vi "Servo_serial_mac_readwrite2.vi"() -> ()   [LabVIEW 2017]
uses:
  <vilib>/Instr/_visa.llb/VISA Configure Serial Port (Instr).vi
panel:
  out "Servo 5 Torque":cluster{i32, dbl, dbl[]}(graph)
  out "Servo 4 Torque":cluster{i32, dbl, dbl[]}(graph)
  out "Servo 3 Torque":cluster{i32, dbl, dbl[]}(graph)
  out "Servo 2 Torque":cluster{i32, dbl, dbl[]}(graph)
  out "Servo 1 Torque":cluster{i32, dbl, dbl[]}(graph)
  out "case offset":i32
  out "case":string
  out "Torq5 number":dbl
  out "Torq4 number":dbl
  out "Torq3 number":dbl
  out "Torq2 number":dbl
  out "Torq1 number":dbl
  out "Servo 5 Position":cluster{i32, dbl, dbl[][]}(graph)
  out "Servo 4 Position":cluster{i32, dbl, dbl[][]}(graph)
  out "Servo 3 Position":cluster{i32, dbl, dbl[][]}(graph)
  out "Servo 2 Position":cluster{i32, dbl, dbl[][]}(graph)
  out "Servo 1 Position":cluster{i32, dbl, dbl[][]}(graph)
  out "Pos1 number":dbl
  out "Pos2 number":dbl
  out "Pos3 number":dbl
  out "Pos4 number":dbl
  out "Pos5 number":dbl
  in  "Delay":dbl
  in  "Buad Rate":i32(ring) items=["2400"=2400, "4800"=4800, "9600"=9600, "14400"=14400, "19200"=19200, "28800"=28800, "38400"=38400, "57600"=57600, "115200"=115200]
  out "Bytes at port":cluster{i32, dbl, dbl[]}(graph)
  out "Read Buffer":string
  in  "Servo 5":dbl(knob) scale=0.0..180.0
  in  "Servo 4":dbl(knob) scale=0.0..180.0
  in  "Servo 3":dbl(knob) scale=0.0..180.0
  in  "Servo 2":dbl(knob) scale=0.0..180.0
  in  "Servo 1":dbl(knob) scale=0.0..180.0
  in  "stop":bool
  out "Sent to Arduino":string
  in  "COM Port":refnum<visa-resource-name>
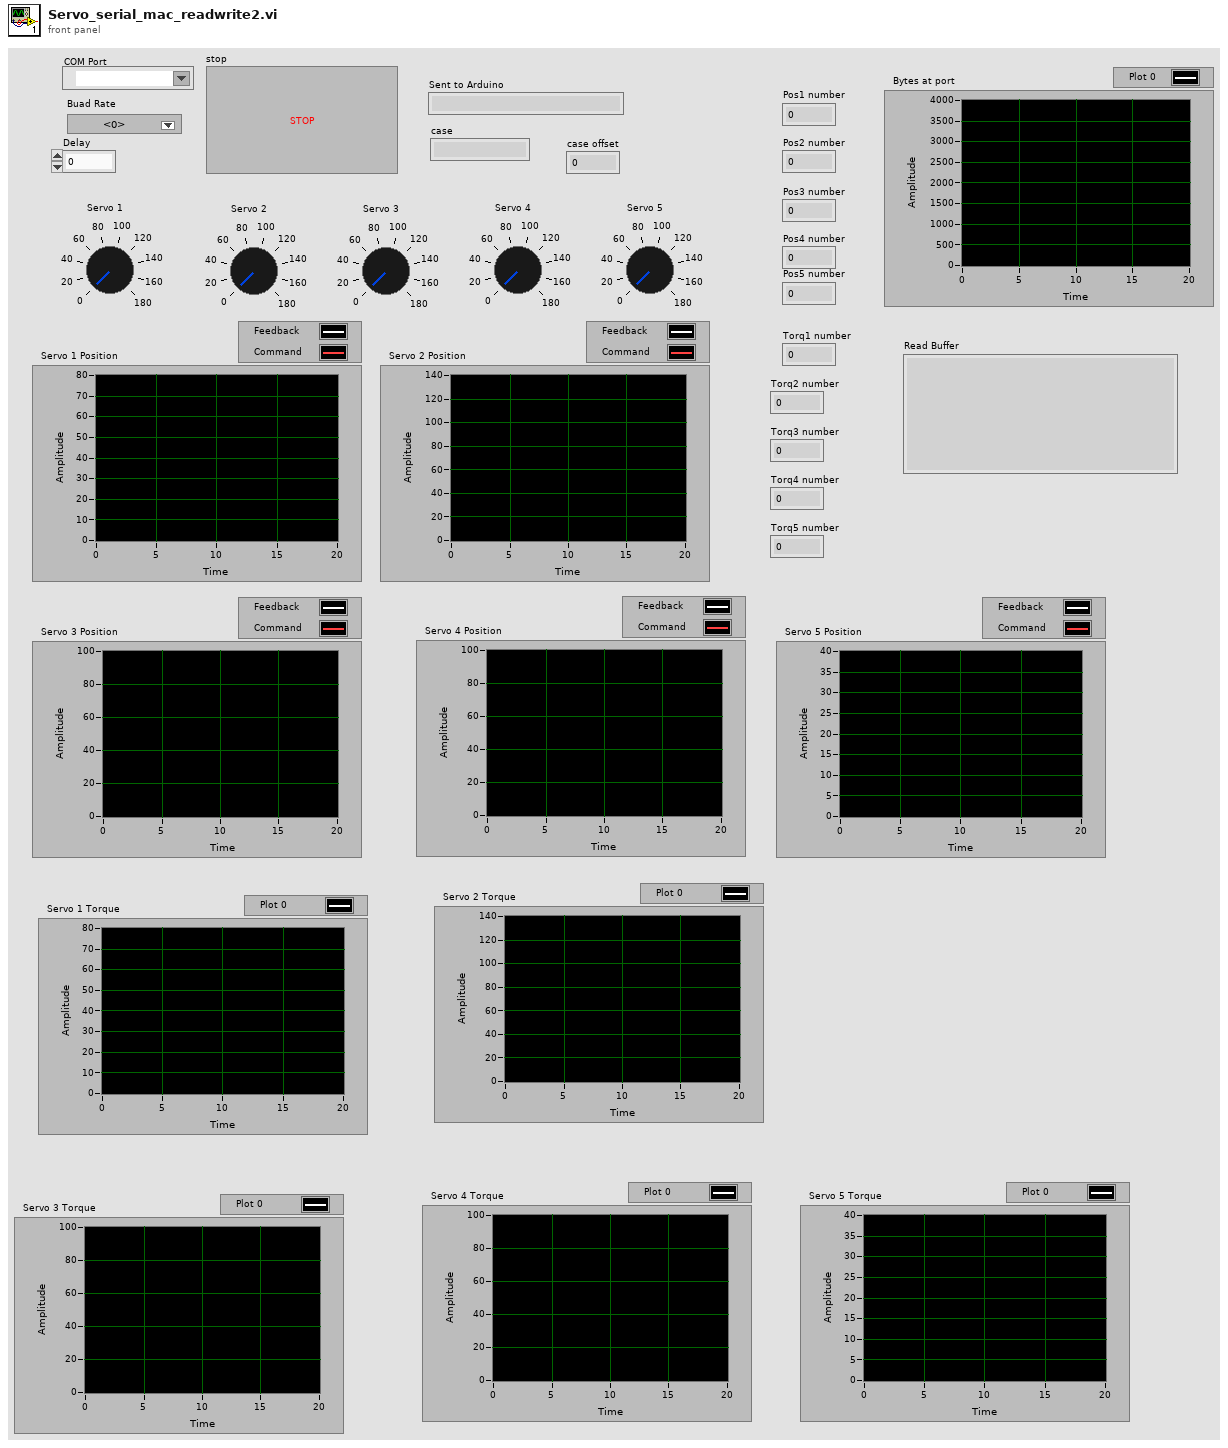
[diagram p1: front panel]
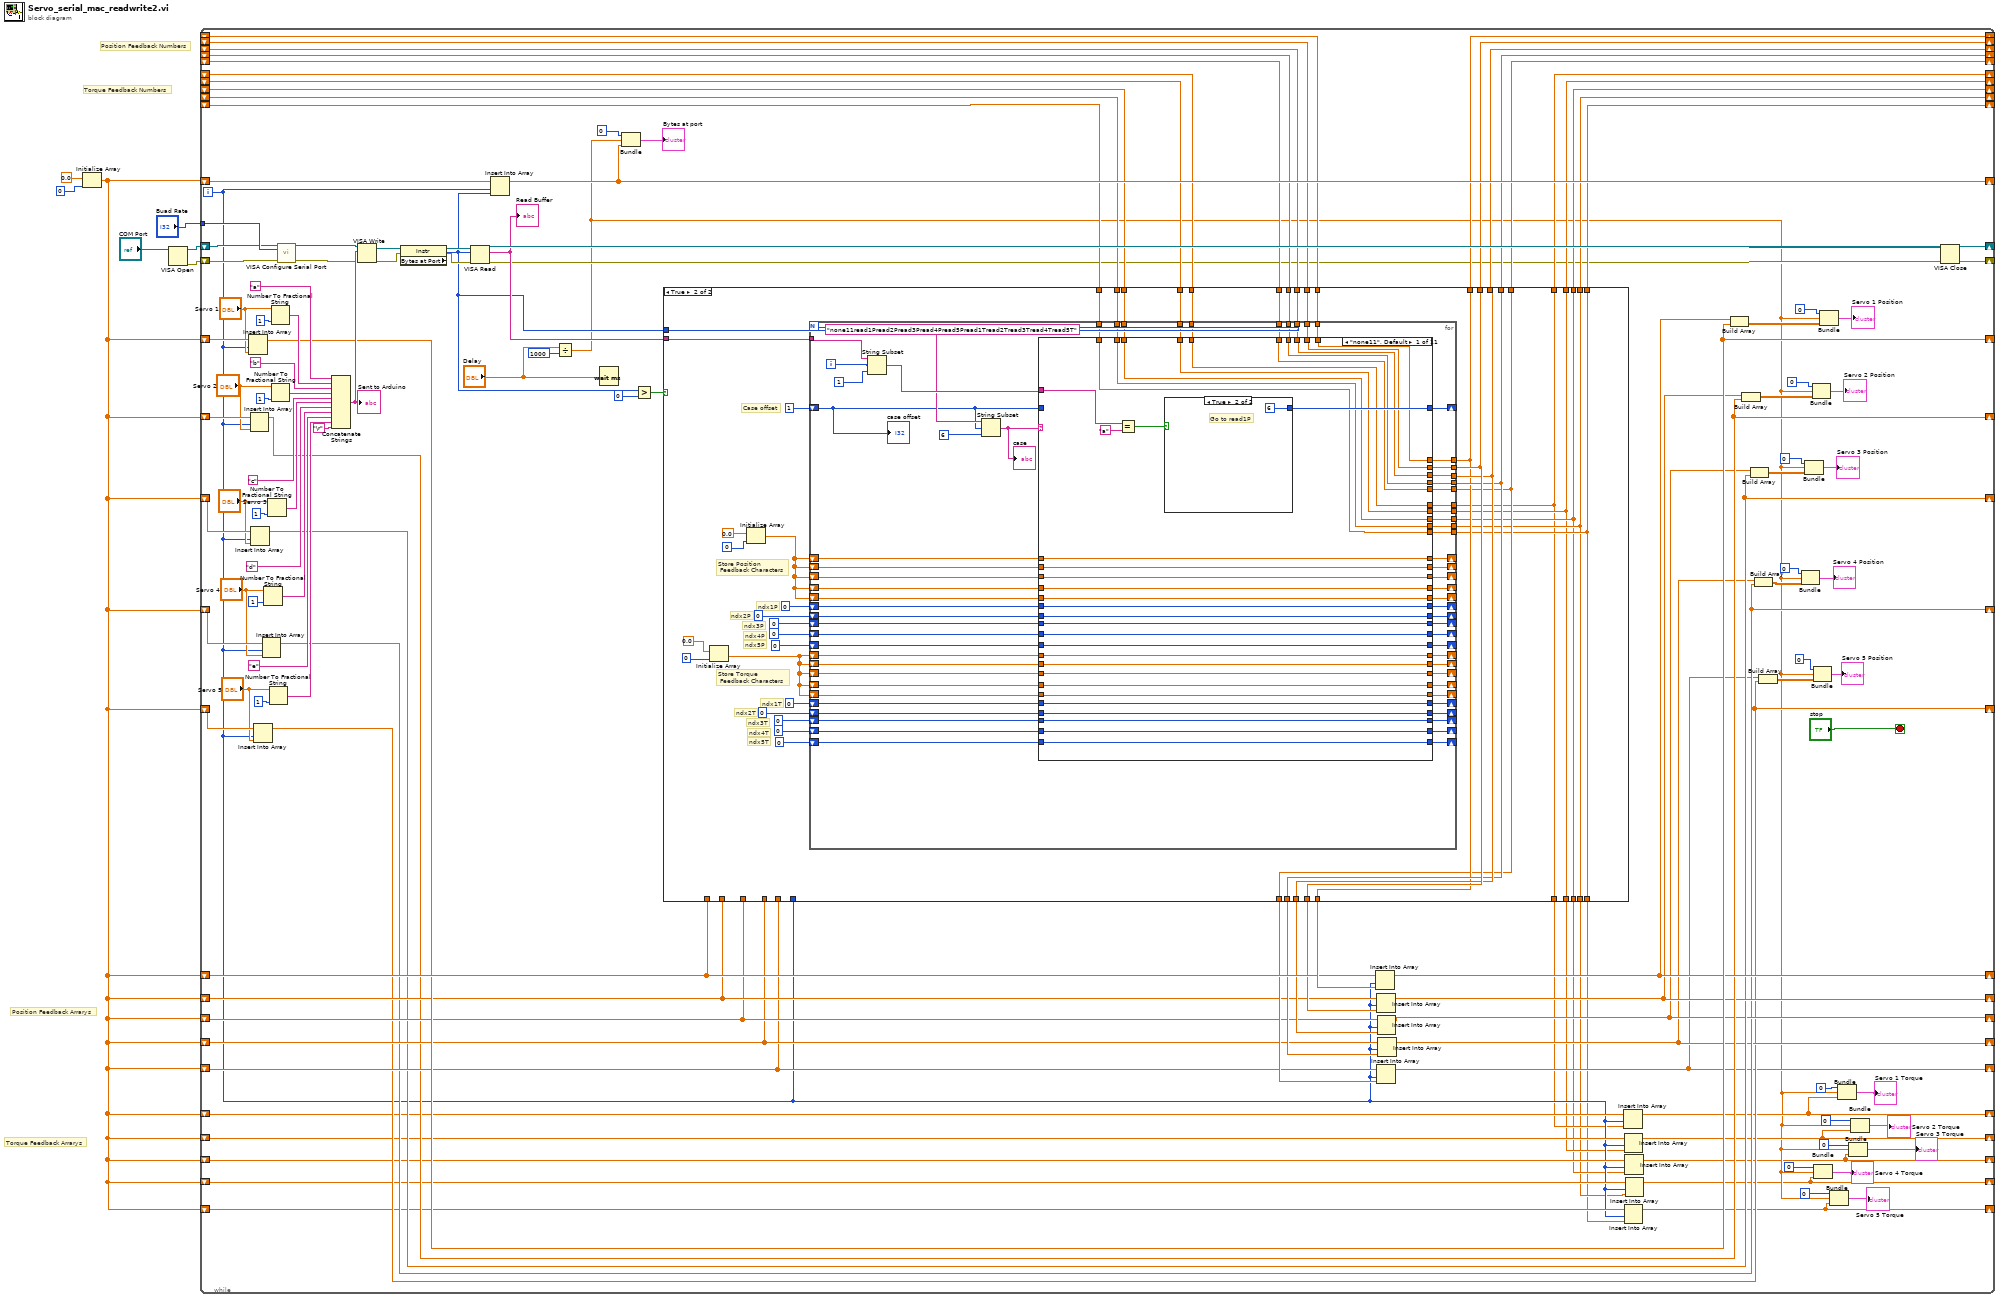
[diagram p0: block diagram]
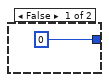
[diagram p3: hidden frame]
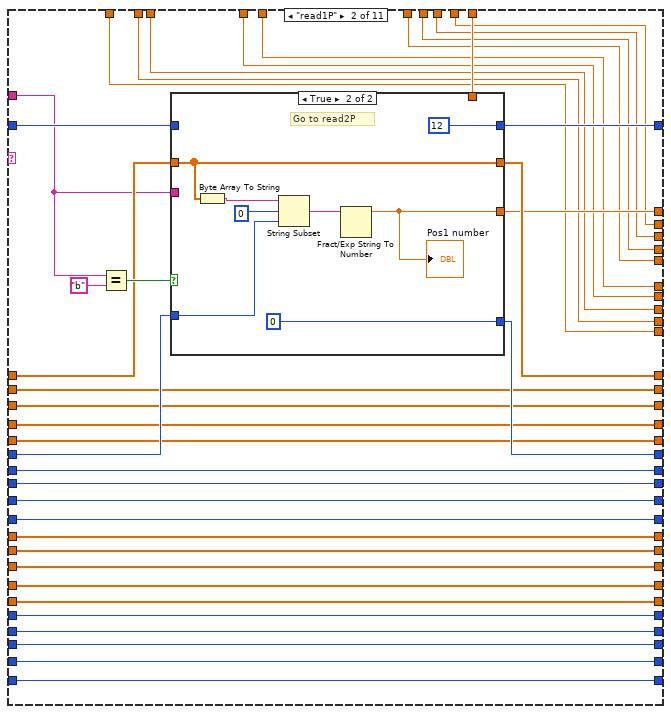
[diagram p4: hidden frame]
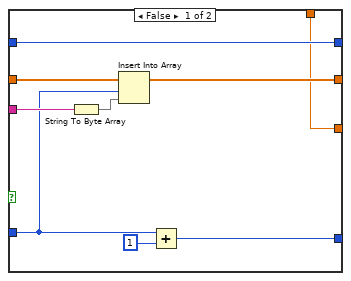
[diagram p5: hidden frame]
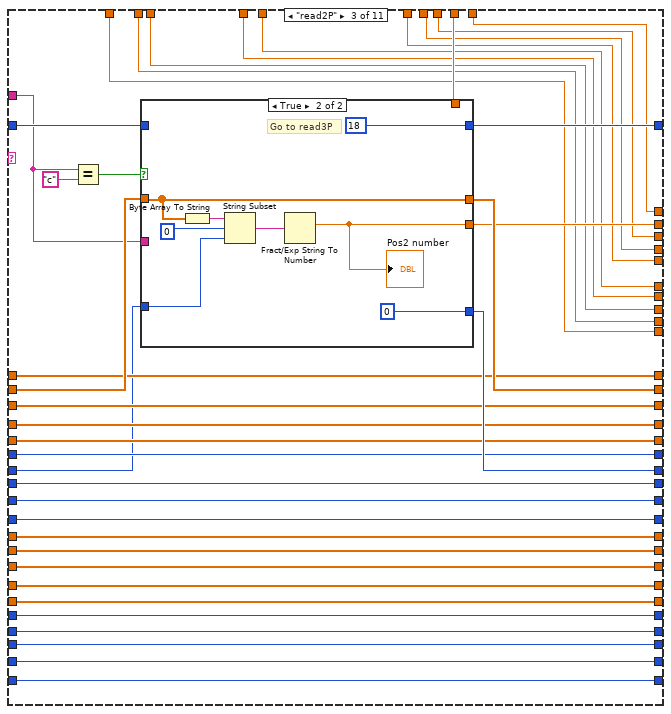
[diagram p6: hidden frame]
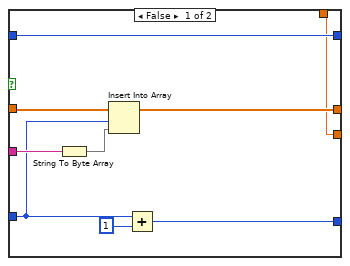
[diagram p7: hidden frame]
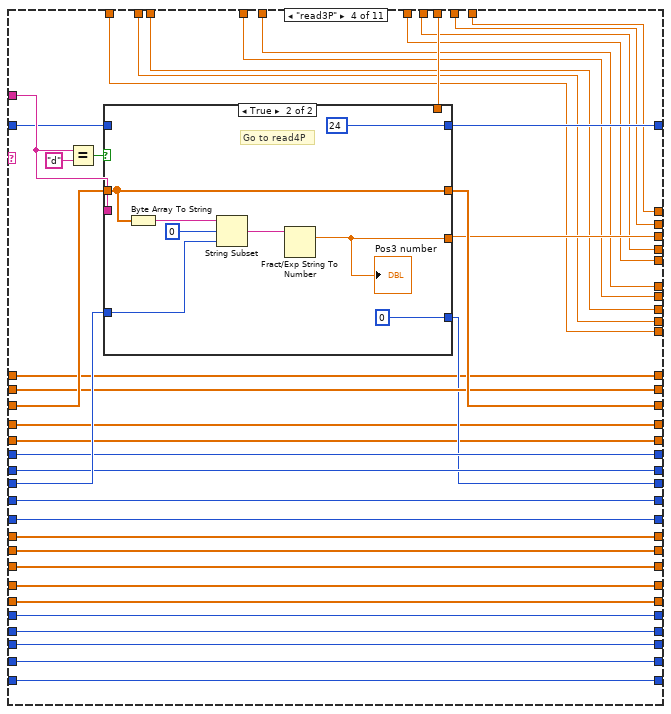
[diagram p8: hidden frame]
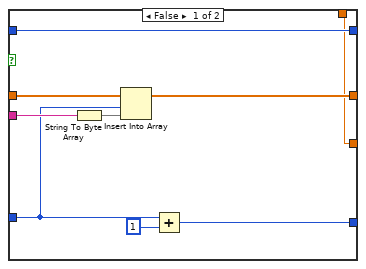
[diagram p9: hidden frame]
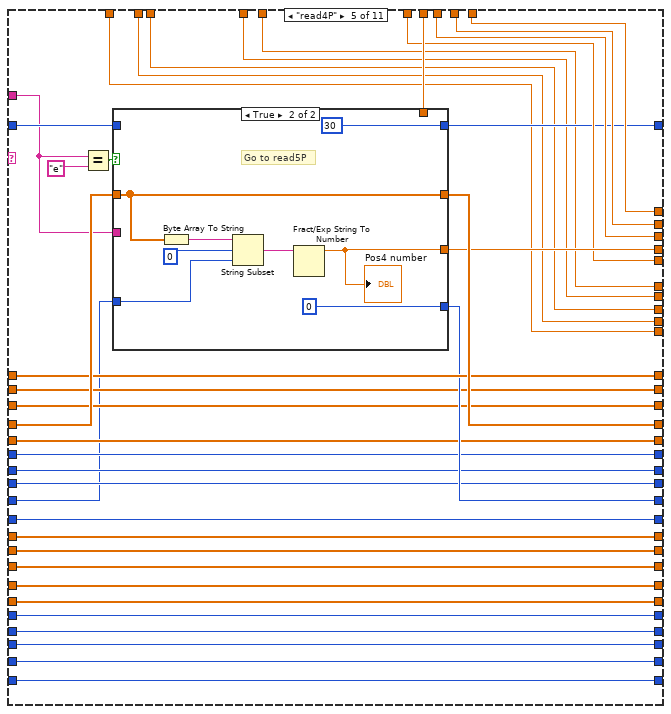
[diagram p10: hidden frame]
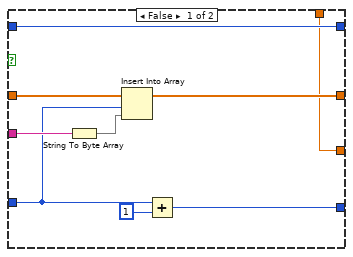
[diagram p11: hidden frame]
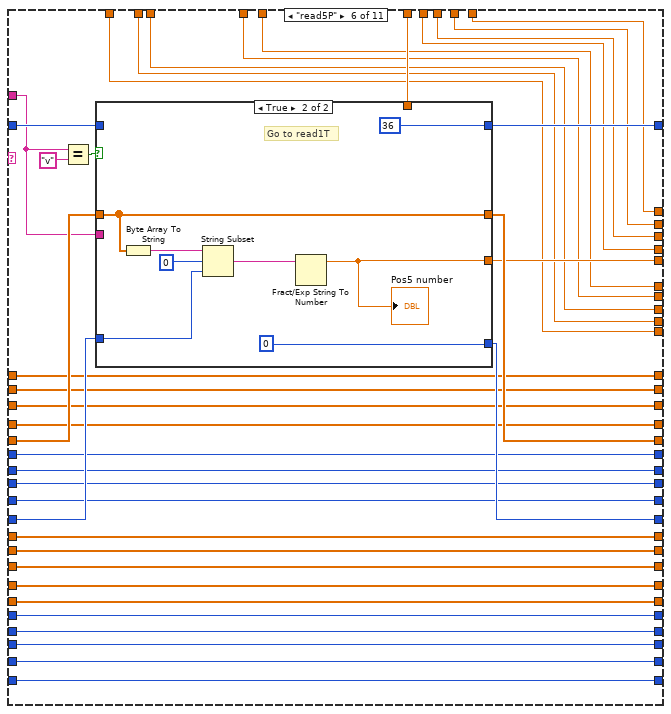
[diagram p12: hidden frame]
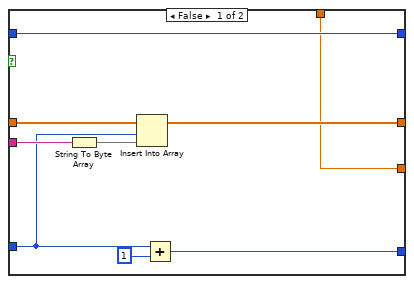
[diagram p13: hidden frame]
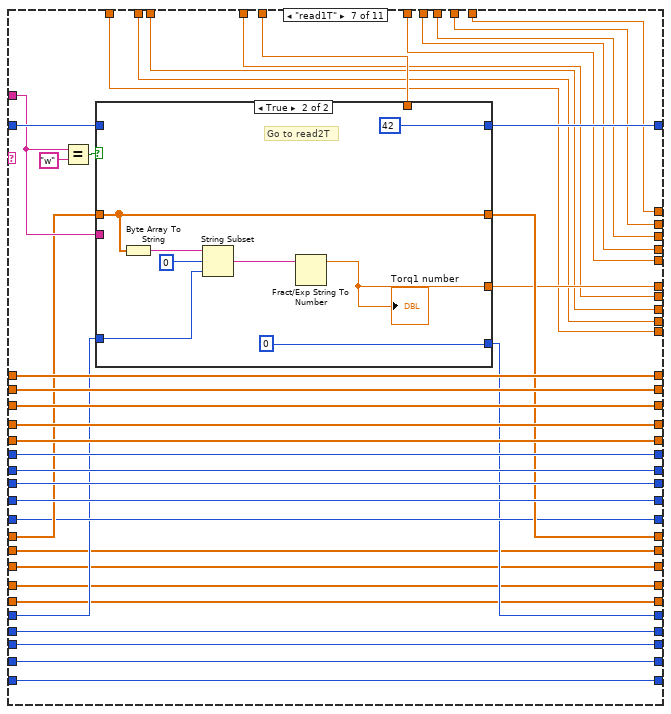
[diagram p14: hidden frame]
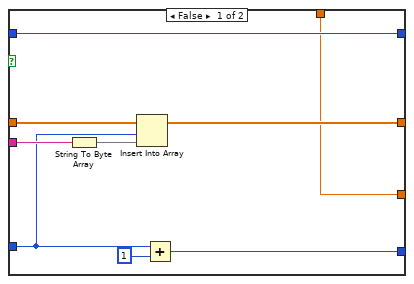
[diagram p15: hidden frame]
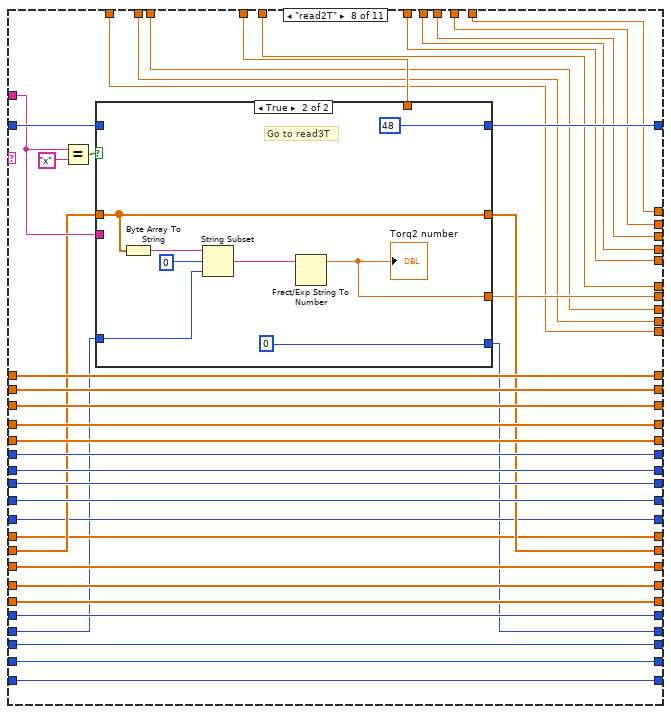
[diagram p16: hidden frame]
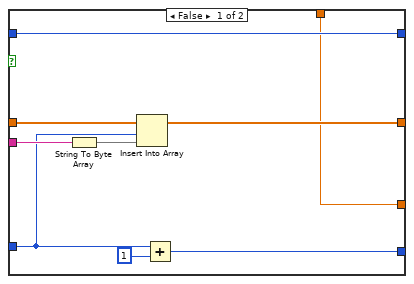
[diagram p17: hidden frame]
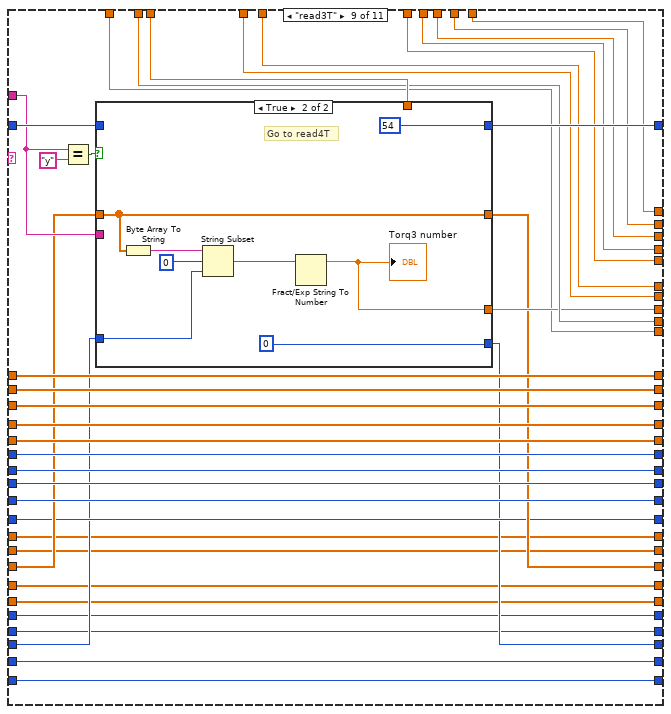
[diagram p18: hidden frame]
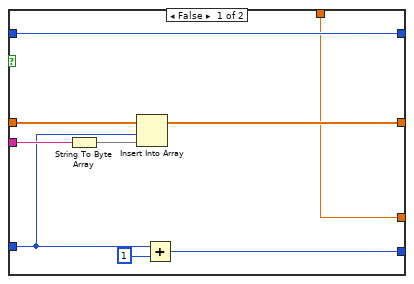
[diagram p19: hidden frame]
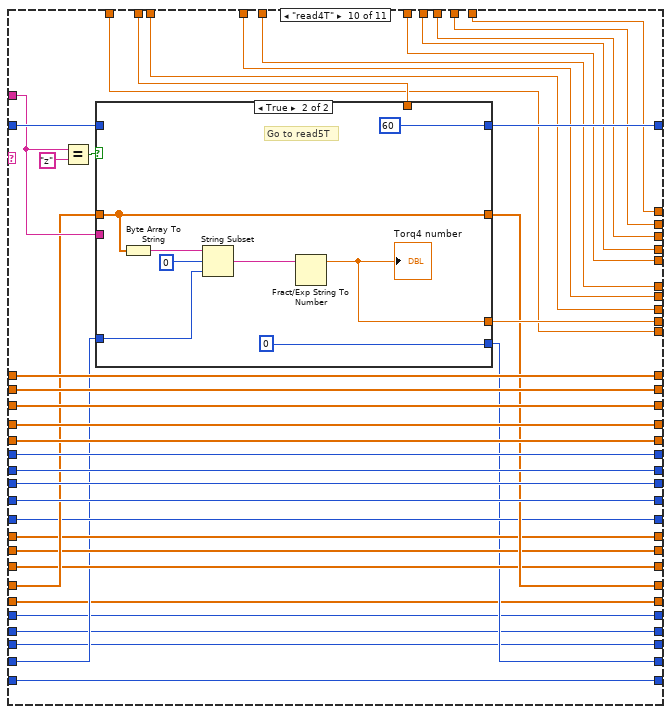
[diagram p20: hidden frame]
diagram:
  # "Torque Feedback Numbers"
  # "Position Feedback Numbers"
  # "Torque Feedback Arrarys"
  # "Position Feedback Arrarys"
  n1 = Initialize Array(0.0 ("element"), 0 ("dimension size")) -> (w1:dbl[])
  n2 = VISA Open(VISA resource name="COM Port") -> (VISA resource name=w8:refnum<visa-resource-name>, error out=w7:errorcluster)  [unwired: 4 in]
  n3 = while {
    tunnel: "Buad Rate" -> [w140]
    shift-right: [w137] -> w6
    shift-left: w8 -> [w139]
    shift-right: [w26] -> w5
    shift-left: w7 -> [w138]
    shift-right: [w135] -> _
    shift-left: w1 -> [w136]
    shift-right: [w81] -> _
    shift-left: w1 -> [w103]
    shift-right: [w69] -> _
    shift-left: w1 -> [w102]
    shift-right: [w66] -> _
    shift-left: w1 -> [w101]
    shift-right: [w63] -> _
    shift-left: w1 -> [w100]
    shift-right: [w60] -> _
    shift-left: w1 -> [w99]
    shift-right: [w79] -> _
    shift-left: w1 -> [w82]
    shift-right: [w68] -> _
    shift-left: w1 -> [w74]
    shift-right: [w65] -> _
    shift-left: w1 -> [w73]
    shift-right: [w62] -> _
    shift-left: w1 -> [w72]
    shift-right: [w59] -> _
    shift-left: w1 -> [w71]
    shift-right: [w49] -> _
    shift-left: _ -> [w58]
    shift-right: [w54] -> _
    shift-left: _ -> [w50]
    shift-right: [w53] -> _
    shift-left: _ -> [w57]
    shift-right: [w52] -> _
    shift-left: _ -> [w56]
    shift-right: [w51] -> _
    shift-left: _ -> [w55]
    shift-right: [w43] -> _
    shift-left: _ -> [w44]
    shift-right: [w42] -> _
    shift-left: _ -> [w45]
    shift-right: [w41] -> _
    shift-left: _ -> [w46]
    shift-right: [w40] -> _
    shift-left: _ -> [w47]
    shift-right: [w39] -> _
    shift-left: _ -> [w48]
    shift-right: [w23] -> _
    shift-left: w1 -> [w38]
    shift-right: [w20] -> _
    shift-left: w1 -> [w37]
    shift-right: [w10] -> _
    shift-left: w1 -> [w36]
    shift-right: [w12] -> _
    shift-left: w1 -> [w35]
    shift-right: [w11] -> _
    shift-left: w1 -> [w34]
    i -> [w33]
    stop <- "stop" stop-if-true
    n4 = Insert Into Array(array=w103, index=w33, new element="Servo 1") -> (w81:dbl[])
    n5 = Insert Into Array(array=w102, index=w33, new element="Servo 2") -> (w69:dbl[])
    n6 = Insert Into Array(array=w101, index=w33, new element="Servo 3") -> (w66:dbl[])
    n7 = Insert Into Array(array=w99, index=w33, new element="Servo 5") -> (w60:dbl[])
    n8 = Insert Into Array(array=w100, index=w33, new element="Servo 4") -> (w63:dbl[])
    n9 = Number To Fractional String(number="Servo 4", precision (6)=1) -> (F-format string=w122:string)  [unwired: 2 in]
    n10 = Number To Fractional String(number="Servo 3", precision (6)=1) -> (F-format string=w129:string)  [unwired: 2 in]
    n11 = Number To Fractional String(number="Servo 5", precision (6)=1) -> (F-format string=w121:string)  [unwired: 2 in]
    n12 = Number To Fractional String(number="Servo 1", precision (6)=1) -> (F-format string=w131:string)  [unwired: 2 in]
    n13 = Number To Fractional String(number="Servo 2", precision (6)=1) -> (F-format string=w130:string)  [unwired: 2 in]
    n14 = call-poly "VISA Configure Serial Port"("VISA resource name"=w139, "baud rate (9600)"=w140, "error in (no error)"=w138) -> ("VISA resource name out"=w120:refnum<visa-resource-name>, "error out"=w132:errorcluster)  [unwired: 11 in]
    n15 = Concatenate Strings("a", w131, "b", w130, "c", w129, "d", w122, "e", w121, "\r") -> (w133:string)
    "Sent to Arduino" <- w133
    n16 = VISA Write(VISA resource name=w120, write buffer=w133, error in (no error)=w132) -> (VISA resource name out=w116:refnum<visa-resource-name>, error out=w119:errorcluster)  [unwired: 1 out]
    n17 = property class="Instr"(reference=w116, error in=w119) -> (reference out=w117:refnum<visa-resource-name>, error out=w118:errorcluster, "Bytes at Port"=w110:u32)
    n18 = VISA Read(VISA resource name=w117, byte count=w110, error in (no error)=w118) -> (VISA resource name out=w137:refnum<visa-resource-name>, read buffer=w112:string, error out=w26:errorcluster)  [unwired: 1 out]
    "Read Buffer" <- w112
    n19 = Insert Into Array(array=w136, index=w33, new element=w110) -> (w135:dbl[])
    n20 = Divide(x="Delay", y=1000) -> (x/y=w13:dbl)
    n21 = Wait (ms)(milliseconds to wait="Delay") -> ()  [unwired: 1 out]
    n22 = Bundle(0, w13, w135) -> (→"Bytes at port":cluster{i32, dbl, dbl[]})  [unwired: 1 in]
    n23 = Greater?(x=w110, y=0) -> (0:w27:bool)
    n24 = case shown="True" w27 {
      tunnel: w110 -> [_ w180]
      tunnel: w112 -> [_ w189]
      tunnel: [w150 w171] -> w83
      tunnel: w33 -> [_ _]
      tunnel: w82 -> [_ _]
      tunnel: [w149 w176] -> w78
      tunnel: [w148 w175] -> w77
      tunnel: [w147 w174] -> w76
      tunnel: [w146 w170] -> w75
      tunnel: w74 -> [_ _]
      tunnel: w73 -> [_ _]
      tunnel: w72 -> [_ _]
      tunnel: w71 -> [_ _]
      tunnel: w58 -> [w150 w179]
      tunnel: w50 -> [w149 w178]
      tunnel: w57 -> [w148 w177]
      tunnel: w56 -> [w147 w173]
      tunnel: w55 -> [w146 w172]
      tunnel: [w150 w171] -> w49
      tunnel: [w149 w176] -> w54
      tunnel: [w148 w175] -> w53
      tunnel: [w147 w174] -> w52
      tunnel: [w146 w170] -> w51
      tunnel: w48 -> [w141 w169]
      tunnel: w47 -> [w142 w168]
      tunnel: w46 -> [w143 w167]
      tunnel: w45 -> [w144 w166]
      tunnel: w44 -> [w145 w165]
      tunnel: [w145 w160] -> w43
      tunnel: [w144 w161] -> w42
      tunnel: [w143 w162] -> w41
      tunnel: [w142 w163] -> w40
      tunnel: [w141 w164] -> w39
      tunnel: [w145 w160] -> w32
      tunnel: [w144 w161] -> w31
      tunnel: [w143 w162] -> w30
      tunnel: [w142 w163] -> w29
      tunnel: [w141 w164] -> w28
      frame False {
      }
      frame True {
        # "Store Torque\n Feedback Characters"
        # "ndx5T"
        # "ndx4T"
        # "ndx3T"
        # "ndx2T"
        # "ndx1T"
        # "Store Position\n Feedback Characters"
        # "ndx5P"
        # "ndx4P"
        # "ndx3P"
        # "ndx2P"
        # "ndx1P"
        # "Case offset"
        n25 = Initialize Array(0.0 ("element"), 0 ("dimension size")) -> (w157:dbl[])
        n26 = Initialize Array(0.0 ("element"), 0 ("dimension size")) -> (w183:dbl[])
        n27 = for {
          N: w180 -> [_]
          tunnel: w189 -> [w257]
          shift-right: [w255] -> _
          shift-left: 1 -> [w190]
          shift-right: [w254] -> _
          shift-left: 0 -> [w253]
          shift-right: [w251] -> _
          shift-left: w183 -> [w252]
          shift-right: [w249] -> _
          shift-left: w183 -> [w250]
          shift-right: [w245] -> _
          shift-left: 0 -> [w248]
          shift-right: [w246] -> _
          shift-left: 0 -> [w247]
          shift-right: [w243] -> _
          shift-left: w183 -> [w244]
          shift-right: [w235] -> _
          shift-left: w183 -> [w242]
          shift-right: [w236] -> _
          shift-left: w183 -> [w241]
          shift-right: [w239] -> _
          shift-left: 0 -> [w240]
          shift-right: [w237] -> _
          shift-left: 0 -> [w238]
          tunnel: w179 -> [w225]
          tunnel: [w234] -> w171
          tunnel: w178 -> [w232]
          tunnel: [w233] -> w176
          tunnel: w177 -> [w230]
          tunnel: [w231] -> w175
          tunnel: w173 -> [w228]
          tunnel: [w229] -> w174
          tunnel: w172 -> [w226]
          tunnel: [w227] -> w170
          tunnel: w169 -> [w223]
          tunnel: w168 -> [w222]
          tunnel: w167 -> [w221]
          tunnel: w166 -> [w220]
          tunnel: w165 -> [w219]
          tunnel: [w218] -> w160
          tunnel: [w217] -> w161
          tunnel: [w216] -> w162
          tunnel: [w215] -> w163
          tunnel: [w214] -> w164
          shift-right: [w212] -> _
          shift-left: w157 -> [w213]
          shift-right: [w211] -> _
          shift-left: w157 -> [w210]
          shift-right: [w209] -> _
          shift-left: w157 -> [w208]
          shift-right: [w207] -> _
          shift-left: w157 -> [w206]
          shift-right: [w205] -> _
          shift-left: w157 -> [w204]
          shift-right: [w203] -> _
          shift-left: 0 -> [w202]
          shift-right: [w201] -> _
          shift-left: 0 -> [w200]
          shift-right: [w199] -> _
          shift-left: 0 -> [w198]
          shift-right: [w196] -> _
          shift-left: 0 -> [w197]
          shift-right: [w195] -> _
          shift-left: 0 -> [w194]
          i -> [w191]
          n28 = String Subset(string=w257, offset (0)=w191, length (rest)=1 ("length (rest)")) -> (substring=w224:string)
          n29 = String Subset(string="none11read1Pread2Pread3Pread4Pread5Pread1Tread2Tread3Tread4Tread5T", offset (0)=w190, length (rest)=6 ("length (rest)")) -> (substring=w193:string)
          "case" <- w193
          n30 = case shown="\"none11\", Default" w193 {
            tunnel: w224 -> [w292 w326 w378 w428 w491 w546 w603 w658 w713 w768 w823]
            tunnel: [w289 w329 w380 w435 w476 w549 w606 w661 w716 w771 w826] -> w255
            tunnel: [w288 w324 w382 w440 w489 w539 w598 w653 w708 w763 w818] -> w254
            tunnel: w253 -> [w288 w325 w382 w440 w489 w539 w598 w653 w708 w763 w818]
            tunnel: w252 -> [w285 w327 w377 w423 w495 w543 w602 w657 w712 w767 w822]
            tunnel: [w285 w330 w377 w423 w495 w543 w602 w657 w712 w767 w822] -> w251
            tunnel: w250 -> [w286 w323 w387 w436 w487 w542 w601 w656 w711 w766 w821]
            tunnel: [w286 w323 w386 w436 w487 w542 w601 w656 w711 w766 w821] -> w249
            tunnel: w248 -> [w287 w319 w365 w439 w488 w538 w597 w652 w707 w762 w817]
            tunnel: [w287 w319 w385 w439 w488 w538 w597 w652 w707 w762 w817] -> w245
            tunnel: w190 -> [_ w328 w381 w420 w492 w548 w605 w660 w715 w770 w825]
            tunnel: w247 -> [w282 w318 w379 w441 w484 w537 w596 w651 w706 w761 w816]
            tunnel: [w282 w318 w379 w432 w484 w537 w596 w651 w706 w761 w816] -> w246
            tunnel: w244 -> [w279 w322 w376 w438 w486 w541 w600 w655 w710 w765 w820]
            tunnel: [w279 w322 w376 w437 w486 w541 w600 w655 w710 w765 w820] -> w243
            tunnel: w242 -> [w280 w321 w375 w431 w497 w540 w599 w654 w709 w764 w819]
            tunnel: w241 -> [w281 w320 w374 w430 w485 w551 w590 w645 w693 w748 w803]
            tunnel: w240 -> [w284 w317 w373 w434 w475 w536 w595 w650 w705 w760 w815]
            tunnel: [w284 w317 w373 w434 w490 w536 w595 w650 w705 w760 w815] -> w239
            tunnel: w238 -> [w283 w316 w372 w433 w483 w545 w587 w634 w690 w742 w800]
            tunnel: [w283 w316 w372 w433 w483 w544 w587 w634 w690 w742 w800] -> w237
            tunnel: [w281 w320 w374 w430 w485 w550 w590 w645 w693 w748 w803] -> w236
            tunnel: [w280 w321 w375 w431 w496 w540 w599 w654 w709 w764 w819] -> w235
            tunnel: [w274 w315 w369 w421 w478 w535 w594 w649 w704 w759 w814] -> w234
            tunnel: w225 -> [w274 w314 w369 w421 w478 w535 w594 w649 w704 w759 w814]
            tunnel: [w278 w313 w371 w427 w482 w530 w591 w646 w701 w756 w811] -> w233
            tunnel: w232 -> [w278 w313 w370 w427 w482 w530 w591 w646 w701 w756 w811]
            tunnel: [w277 w312 w366 w426 w479 w533 w593 w648 w703 w758 w813] -> w231
            tunnel: w230 -> [w277 w312 w366 w425 w479 w533 w593 w648 w703 w758 w813]
            tunnel: [w276 w311 w368 w424 w481 w531 w592 w647 w702 w757 w812] -> w229
            tunnel: w228 -> [w276 w311 w368 w424 w480 w531 w592 w647 w702 w757 w812]
            tunnel: [w275 w310 w367 w422 w477 w534 w583 w629 w699 w755 w810] -> w227
            tunnel: w226 -> [w275 w310 w367 w422 w477 w532 w583 w629 w699 w755 w810]
            tunnel: w223 -> [w269 w305 w360 w415 w470 w525 w571 w625 w694 w749 w809]
            tunnel: w222 -> [w270 w306 w361 w416 w471 w526 w572 w626 w696 w754 w804]
            tunnel: w221 -> [w271 w307 w362 w417 w472 w527 w573 w627 w700 w751 w805]
            tunnel: w220 -> [w272 w308 w363 w418 w473 w528 w574 w631 w697 w752 w806]
            tunnel: w219 -> [w273 w309 w364 w419 w474 w529 w584 w630 w698 w753 w807]
            tunnel: [w273 w309 w364 w419 w474 w529 w582 w630 w698 w753 w807] -> w218
            tunnel: [w272 w308 w363 w418 w473 w528 w574 w628 w697 w752 w806] -> w217
            tunnel: [w271 w307 w362 w417 w472 w527 w573 w627 w695 w751 w805] -> w216
            tunnel: [w270 w306 w361 w416 w471 w526 w572 w626 w696 w750 w804] -> w215
            tunnel: [w269 w305 w360 w415 w470 w525 w571 w625 w694 w749 w808] -> w214
            tunnel: w213 -> [w268 w304 w359 w414 w469 w524 w589 w642 w687 w745 w790]
            tunnel: [w268 w304 w359 w414 w469 w524 w588 w642 w687 w745 w790] -> w212
            tunnel: [w267 w303 w358 w413 w468 w523 w581 w643 w686 w744 w791] -> w211
            tunnel: w210 -> [w267 w303 w358 w413 w468 w523 w581 w644 w686 w744 w791]
            tunnel: [w266 w302 w357 w412 w467 w522 w580 w641 w691 w743 w792] -> w209
            tunnel: w208 -> [w266 w302 w357 w412 w467 w522 w580 w641 w692 w743 w792]
            tunnel: [w265 w301 w356 w411 w466 w521 w579 w640 w685 w747 w793] -> w207
            tunnel: w206 -> [w265 w301 w356 w411 w466 w521 w579 w640 w685 w746 w793]
            tunnel: [w264 w300 w355 w410 w465 w520 w578 w639 w684 w738 w802] -> w205
            tunnel: w204 -> [w264 w300 w355 w410 w465 w520 w578 w639 w684 w738 w801]
            tunnel: [w263 w299 w354 w409 w464 w519 w585 w638 w683 w739 w794] -> w203
            tunnel: w202 -> [w263 w299 w354 w409 w464 w519 w586 w638 w683 w739 w794]
            tunnel: [w262 w298 w353 w408 w463 w518 w577 w633 w682 w737 w795] -> w201
            tunnel: w200 -> [w262 w298 w353 w408 w463 w518 w577 w632 w682 w737 w795]
            tunnel: [w261 w297 w352 w407 w462 w517 w576 w637 w689 w736 w796] -> w199
            tunnel: w198 -> [w261 w297 w352 w407 w462 w517 w576 w637 w688 w736 w796]
            tunnel: w197 -> [w260 w296 w351 w406 w461 w516 w575 w636 w681 w740 w797]
            tunnel: [w260 w296 w351 w406 w461 w516 w575 w636 w681 w741 w797] -> w196
            tunnel: [w259 w295 w350 w405 w460 w515 w570 w635 w680 w735 w799] -> w195
            tunnel: w194 -> [w259 w295 w350 w405 w460 w515 w570 w635 w680 w735 w798]
            frame "none11", Default {
              n31 = Equal?(x=w292, y="a") -> (x = y?=w290:bool)
              n32 = case shown="True" w290 {
                tunnel: [0 6] -> w289
                frame False {
                }
                frame True {
                  # "Go to read1P"
                }
              }
            }
            frame "read1P" {
              n33 = Equal?(x=w326, y="b") -> (x = y?=w331:bool)
              n34 = case shown="True" w331 {
                tunnel: [w341 0] -> w324
                tunnel: w327 -> [w335 w345]
                tunnel: [w339 w345] -> w330
                tunnel: w326 -> [w338 _]
                tunnel: [w336 12] -> w329
                tunnel: w328 -> [w336 _]
                tunnel: w325 -> [w334 w344]
                tunnel: [w333 w342] -> w315
                tunnel: w314 -> [w333 _]
                frame False {
                  n35 = String To Byte Array(string=w338) -> (unsigned byte array=w337:u8[])
                  n36 = Insert Into Array(array=w335, index=w334, new element=w337) -> (w339:dbl[])
                  n37 = Add(x=w334, y=1) -> (x+y=w341:i32)
                }
                frame True {
                  # "Go to read2P"
                  n38 = Byte Array To String(unsigned byte array=w345) -> (string=w346:string)
                  n39 = String Subset(string=w346, offset (0)=0, length (rest)=w344) -> (substring=w343:string)
                  n40 = Fract/Exp String To Number(string=w343) -> (number=w342:dbl)  [unwired: 3 in, 1 out]
                  "Pos1 number" <- w342
                }
              }
            }
            frame "read2P" {
              n41 = Equal?(x=w378, y="c") -> (x = y?=w383:bool)
              n42 = case shown="True" w383 {
                tunnel: [w396 0] -> w385
                tunnel: w365 -> [w390 w401]
                tunnel: w387 -> [w394 w398]
                tunnel: [w393 w398] -> w386
                tunnel: w378 -> [w392 _]
                tunnel: [w389 18] -> w380
                tunnel: w381 -> [w389 _]
                tunnel: [w388 w399] -> w371
                tunnel: w370 -> [w388 _]
                frame False {
                  n43 = String To Byte Array(string=w392) -> (unsigned byte array=w391:u8[])
                  n44 = Insert Into Array(array=w394, index=w390, new element=w391) -> (w393:dbl[])
                  n45 = Add(x=w390, y=1) -> (x+y=w396:i32)
                }
                frame True {
                  # "Go to read3P"
                  n46 = Byte Array To String(unsigned byte array=w398) -> (string=w397:string)
                  n47 = String Subset(string=w397, offset (0)=0, length (rest)=w401) -> (substring=w400:string)
                  n48 = Fract/Exp String To Number(string=w400) -> (number=w399:dbl)  [unwired: 3 in, 1 out]
                  "Pos2 number" <- w399
                }
              }
            }
            frame "read3P" {
              n49 = Equal?(x=w428, y="d") -> (x = y?=w442:bool)
              n50 = case shown="True" w442 {
                tunnel: [w451 0] -> w432
                tunnel: w441 -> [w445 w454]
                tunnel: w438 -> [w449 w455]
                tunnel: [w448 w455] -> w437
                tunnel: w428 -> [w447 _]
                tunnel: [w444 24] -> w435
                tunnel: w420 -> [w444 _]
                tunnel: [w443 w452] -> w426
                tunnel: w425 -> [w443 _]
                frame False {
                  n51 = String To Byte Array(string=w447) -> (unsigned byte array=w446:u8[])
                  n52 = Insert Into Array(array=w449, index=w445, new element=w446) -> (w448:dbl[])
                  n53 = Add(x=w445, y=1) -> (x+y=w451:i32)
                }
                frame True {
                  # "Go to read4P"
                  n54 = Byte Array To String(unsigned byte array=w455) -> (string=w456:string)
                  n55 = String Subset(string=w456, offset (0)=0, length (rest)=w454) -> (substring=w453:string)
                  n56 = Fract/Exp String To Number(string=w453) -> (number=w452:dbl)  [unwired: 3 in, 1 out]
                  "Pos3 number" <- w452
                }
              }
            }
            frame "read4P" {
              n57 = Equal?(x=w491, y="e") -> (x = y?=w493:bool)
              n58 = case shown="True" w493 {
                tunnel: [w506 0] -> w490
                tunnel: w475 -> [w500 w509]
                tunnel: w497 -> [w504 w510]
                tunnel: [w503 w510] -> w496
                tunnel: w491 -> [w502 _]
                tunnel: [w499 30] -> w476
                tunnel: w492 -> [w499 _]
                tunnel: [w498 w507] -> w481
                tunnel: w480 -> [w498 _]
                frame False {
                  n59 = String To Byte Array(string=w502) -> (unsigned byte array=w501:u8[])
                  n60 = Insert Into Array(array=w504, index=w500, new element=w501) -> (w503:dbl[])
                  n61 = Add(x=w500, y=1) -> (x+y=w506:i32)
                }
                frame True {
                  # "Go to read5P"
                  n62 = Byte Array To String(unsigned byte array=w510) -> (string=w511:string)
                  n63 = String Subset(string=w511, offset (0)=0, length (rest)=w509) -> (substring=w508:string)
                  n64 = Fract/Exp String To Number(string=w508) -> (number=w507:dbl)  [unwired: 3 in, 1 out]
                  "Pos4 number" <- w507
                }
              }
            }
            frame "read5P" {
              n65 = Equal?(x=w546, y="v") -> (x = y?=w547:bool)
              n66 = case shown="True" w547 {
                tunnel: [w561 0] -> w544
                tunnel: w545 -> [w555 w562]
                tunnel: w551 -> [w559 w565]
                tunnel: [w558 w565] -> w550
                tunnel: w546 -> [w557 _]
                tunnel: [w554 36] -> w549
                tunnel: w548 -> [w554 _]
                tunnel: [w553 w563] -> w534
                tunnel: w532 -> [w553 _]
                frame False {
                  n67 = String To Byte Array(string=w557) -> (unsigned byte array=w556:u8[])
                  n68 = Insert Into Array(array=w559, index=w555, new element=w556) -> (w558:dbl[])
                  n69 = Add(x=w555, y=1) -> (x+y=w561:i32)
                }
                frame True {
                  # "Go to read1T"
                  n70 = Byte Array To String(unsigned byte array=w565) -> (string=w566:string)
                  n71 = String Subset(string=w566, offset (0)=0, length (rest)=w562) -> (substring=w564:string)
                  n72 = Fract/Exp String To Number(string=w564) -> (number=w563:dbl)  [unwired: 3 in, 1 out]
                  "Pos5 number" <- w563
                }
              }
            }
            frame "read1T" {
              n73 = Equal?(x=w603, y="w") -> (x = y?=w604:bool)
              n74 = case shown="True" w604 {
                tunnel: [w616 0] -> w585
                tunnel: w586 -> [w610 w617]
                tunnel: w589 -> [w614 w620]
                tunnel: [w613 w620] -> w588
                tunnel: w603 -> [w612 _]
                tunnel: [w609 42] -> w606
                tunnel: w605 -> [w609 _]
                tunnel: [w608 w618] -> w582
                tunnel: w584 -> [w608 _]
                frame False {
                  n75 = String To Byte Array(string=w612) -> (unsigned byte array=w611:u8[])
                  n76 = Insert Into Array(array=w614, index=w610, new element=w611) -> (w613:dbl[])
                  n77 = Add(x=w610, y=1) -> (x+y=w616:i32)
                }
                frame True {
                  # "Go to read2T"
                  n78 = Byte Array To String(unsigned byte array=w620) -> (string=w621:string)
                  n79 = String Subset(string=w621, offset (0)=0, length (rest)=w617) -> (substring=w619:string)
                  n80 = Fract/Exp String To Number(string=w619) -> (number=w618:dbl)  [unwired: 3 in, 1 out]
                  "Torq1 number" <- w618
                }
              }
            }
            frame "read2T" {
              n81 = Equal?(x=w658, y="x") -> (x = y?=w659:bool)
              n82 = case shown="True" w659 {
                tunnel: [w671 0] -> w633
                tunnel: w632 -> [w665 w672]
                tunnel: w644 -> [w669 w675]
                tunnel: [w668 w675] -> w643
                tunnel: w658 -> [w667 _]
                tunnel: [w664 48] -> w661
                tunnel: w660 -> [w664 _]
                tunnel: [w663 w673] -> w628
                tunnel: w631 -> [w663 _]
                frame False {
                  n83 = String To Byte Array(string=w667) -> (unsigned byte array=w666:u8[])
                  n84 = Insert Into Array(array=w669, index=w665, new element=w666) -> (w668:dbl[])
                  n85 = Add(x=w665, y=1) -> (x+y=w671:i32)
                }
                frame True {
                  # "Go to read3T"
                  n86 = Byte Array To String(unsigned byte array=w675) -> (string=w676:string)
                  n87 = String Subset(string=w676, offset (0)=0, length (rest)=w672) -> (substring=w674:string)
                  n88 = Fract/Exp String To Number(string=w674) -> (number=w673:dbl)  [unwired: 3 in, 1 out]
                  "Torq2 number" <- w673
                }
              }
            }
            frame "read3T" {
              n89 = Equal?(x=w713, y="y") -> (x = y?=w714:bool)
              n90 = case shown="True" w714 {
                tunnel: [w726 0] -> w689
                tunnel: w688 -> [w720 w727]
                tunnel: w692 -> [w724 w730]
                tunnel: [w723 w730] -> w691
                tunnel: w713 -> [w722 _]
                tunnel: [w719 54] -> w716
                tunnel: w715 -> [w719 _]
                tunnel: [w718 w728] -> w695
                tunnel: w700 -> [w718 _]
                frame False {
                  n91 = String To Byte Array(string=w722) -> (unsigned byte array=w721:u8[])
                  n92 = Insert Into Array(array=w724, index=w720, new element=w721) -> (w723:dbl[])
                  n93 = Add(x=w720, y=1) -> (x+y=w726:i32)
                }
                frame True {
                  # "Go to read4T"
                  n94 = Byte Array To String(unsigned byte array=w730) -> (string=w731:string)
                  n95 = String Subset(string=w731, offset (0)=0, length (rest)=w727) -> (substring=w729:string)
                  n96 = Fract/Exp String To Number(string=w729) -> (number=w728:dbl)  [unwired: 3 in, 1 out]
                  "Torq3 number" <- w728
                }
              }
            }
            frame "read4T" {
              n97 = Equal?(x=w768, y="z") -> (x = y?=w769:bool)
              n98 = case shown="True" w769 {
                tunnel: [w781 0] -> w741
                tunnel: w740 -> [w775 w782]
                tunnel: w746 -> [w779 w785]
                tunnel: [w778 w785] -> w747
                tunnel: w768 -> [w777 _]
                tunnel: [w774 60] -> w771
                tunnel: w770 -> [w774 _]
                tunnel: [w773 w783] -> w750
                tunnel: w754 -> [w773 _]
                frame False {
                  n99 = String To Byte Array(string=w777) -> (unsigned byte array=w776:u8[])
                  n100 = Insert Into Array(array=w779, index=w775, new element=w776) -> (w778:dbl[])
                  n101 = Add(x=w775, y=1) -> (x+y=w781:i32)
                }
                frame True {
                  # "Go to read5T"
                  n102 = Byte Array To String(unsigned byte array=w785) -> (string=w786:string)
                  n103 = String Subset(string=w786, offset (0)=0, length (rest)=w782) -> (substring=w784:string)
                  n104 = Fract/Exp String To Number(string=w784) -> (number=w783:dbl)  [unwired: 3 in, 1 out]
                  "Torq4 number" <- w783
                }
              }
            }
            frame "read5T" {
              n105 = Equal?(x=w823, y="!") -> (x = y?=w824:bool)
              n106 = case shown="True" w824 {
                tunnel: [w836 0] -> w799
                tunnel: w798 -> [w830 w837]
                tunnel: w801 -> [w834 w840]
                tunnel: [w833 w840] -> w802
                tunnel: w823 -> [w832 _]
                tunnel: [w829 0] -> w826
                tunnel: w825 -> [w829 _]
                tunnel: [w828 w838] -> w808
                tunnel: w809 -> [w828 _]
                frame False {
                  n107 = String To Byte Array(string=w832) -> (unsigned byte array=w831:u8[])
                  n108 = Insert Into Array(array=w834, index=w830, new element=w831) -> (w833:dbl[])
                  n109 = Add(x=w830, y=1) -> (x+y=w836:i32)
                }
                frame True {
                  # "Go to none11"
                  n110 = Byte Array To String(unsigned byte array=w840) -> (string=w841:string)
                  n111 = String Subset(string=w841, offset (0)=0, length (rest)=w837) -> (substring=w839:string)
                  n112 = Fract/Exp String To Number(string=w839) -> (number=w838:dbl)  [unwired: 3 in, 1 out]
                  "Torq5 number" <- w838
                }
              }
            }
          }
          "case offset" <- w190
        }
      }
    }
    n113 = Insert Into Array(array=w82, index=w33, new element=w83) -> (w79:dbl[])
    n114 = Insert Into Array(array=w74, index=w33, new element=w78) -> (w68:dbl[])
    n115 = Insert Into Array(array=w71, index=w33, new element=w75) -> (w59:dbl[])
    n116 = Insert Into Array(array=w73, index=w33, new element=w77) -> (w65:dbl[])
    n117 = Insert Into Array(array=w72, index=w33, new element=w76) -> (w62:dbl[])
    n118 = Insert Into Array(array=w38, index=w33, new element=w32) -> (w23:dbl[])
    n119 = Insert Into Array(array=w37, index=w33, new element=w31) -> (w20:dbl[])
    n120 = Insert Into Array(array=w34, index=w33, new element=w28) -> (w11:dbl[])
    n121 = Insert Into Array(array=w36, index=w33, new element=w30) -> (w10:dbl[])
    n122 = Insert Into Array(array=w35, index=w33, new element=w29) -> (w12:dbl[])
    n123 = Build Array(w79, w81) -> (w80:dbl[][])
    n124 = Build Array(w68, w69) -> (w70:dbl[][])
    n125 = Build Array(w65, w66) -> (w67:dbl[][])
    n126 = Build Array(w62, w63) -> (w64:dbl[][])
    n127 = Build Array(w59, w60) -> (w61:dbl[][])
    n128 = Bundle(0, w13, w64) -> (→"Servo 4 Position":cluster{i32, dbl, dbl[][]})  [unwired: 1 in]
    n129 = Bundle(0, w13, w67) -> (→"Servo 3 Position":cluster{i32, dbl, dbl[][]})  [unwired: 1 in]
    n130 = Bundle(0, w13, w70) -> (→"Servo 2 Position":cluster{i32, dbl, dbl[][]})  [unwired: 1 in]
    n131 = Bundle(0, w13, w61) -> (→"Servo 5 Position":cluster{i32, dbl, dbl[][]})  [unwired: 1 in]
    n132 = Bundle(0, w13, w12) -> (→"Servo 4 Torque":cluster{i32, dbl, dbl[]})  [unwired: 1 in]
    n133 = Bundle(0, w13, w80) -> (→"Servo 1 Position":cluster{i32, dbl, dbl[][]})  [unwired: 1 in]
    n134 = Bundle(0, w13, w11) -> (→"Servo 5 Torque":cluster{i32, dbl, dbl[]})  [unwired: 1 in]
    n135 = Bundle(0, w13, w23) -> (→"Servo 1 Torque":cluster{i32, dbl, dbl[]})  [unwired: 1 in]
    n136 = Bundle(0, w13, w10) -> (→"Servo 3 Torque":cluster{i32, dbl, dbl[]})  [unwired: 1 in]
    n137 = Bundle(0, w13, w20) -> (→"Servo 2 Torque":cluster{i32, dbl, dbl[]})  [unwired: 1 in]
  }
  n138 = VISA Close(VISA resource name=w6, error in (no error)=w5) -> ()  [unwired: 1 out]
